vi "Write Source Waveform Task Data Property.vi"(8 "error in (no error)":errorcluster, 10 "Source Waveform Data":T2, 11 "Result Section ref":T1=18446744073709551615 format="%.0x") -> (0 "error out":errorcluster, 3 "Result Section ref out":T1=18446744073709551615 format="%.0x")   [LabVIEW 2015, in "Waveform-Processing-Custom-Device System Explorer.lvlib"]
uses:
  Waveform-Processing-Custom-Device System Explorer.lvlib
  <vilib>/NI Veristand/Custom Device API/Custom Device Item Ref.ctl
  Shared/Constants.vi
  <vilib>/NI Veristand/Custom Device API/Set Item Property (Double).vi
  <vilib>/NI Veristand/Custom Device API/Set Item Property (Boolean).vi
  <vilib>/NI Veristand/Custom Device API/Set Item Property (U32).vi
  <vilib>/NI VeriStand/Custom Device API/Custom Device API.lvlib
  Shared/Waveform-Processing-Custom-Device Shared.lvlib
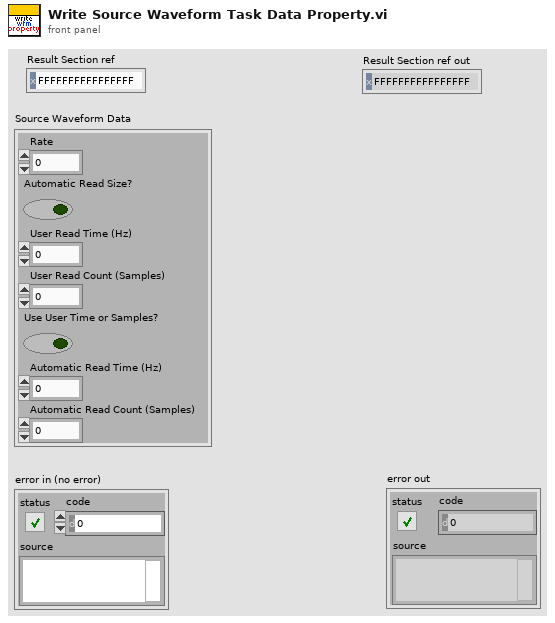
[diagram p1: front panel]
types:
  T1 = typedef "Custom Device API.lvlib/Custom Device Item Ref.ctl" = u64
  T2 = cluster{"Rate":dbl, "Automatic Read Size?":bool, "User Read Time (Hz) ":dbl, "User Read Count (Samples) ":u32, "Use User Time or Samples?":bool, "Automatic Read Time (Hz)":dbl, "Automatic Read Count (Samples)":u32}
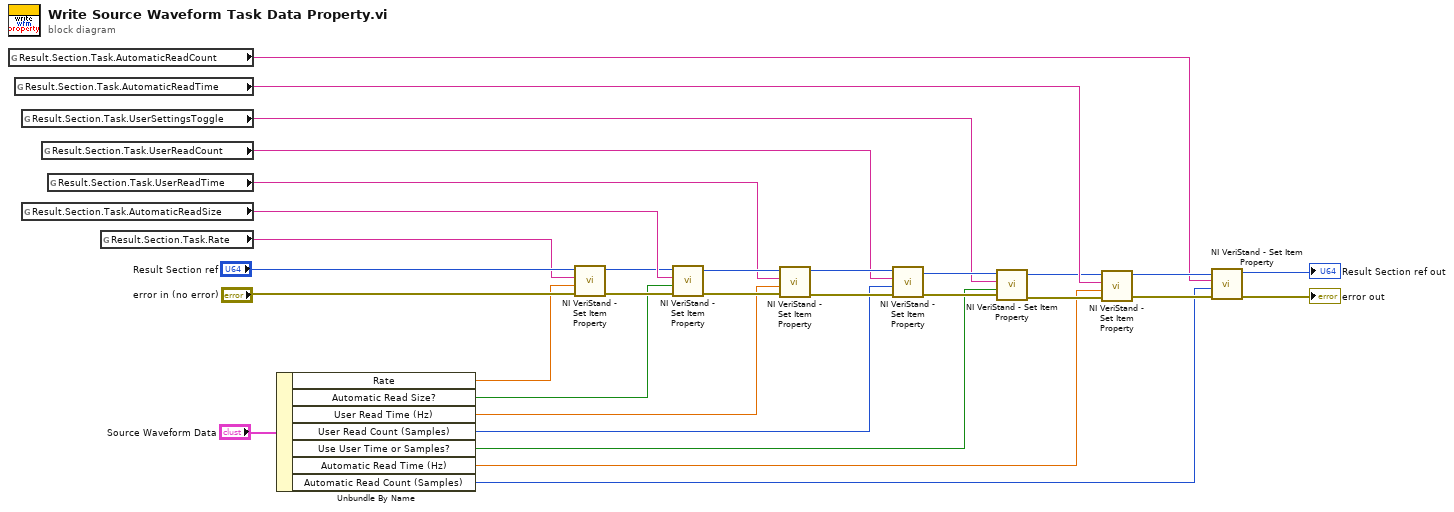
[diagram p0: block diagram]
diagram:
  n1 = global read "Constants.vi" "Result.Section.Task.AutomaticReadCount"() -> (w4:string)
  n2 = global read "Constants.vi" "Result.Section.Task.AutomaticReadTime"() -> (w10:string)
  n3 = global read "Constants.vi" "Result.Section.Task.UserSettingsToggle"() -> (w13:string)
  n4 = global read "Constants.vi" "Result.Section.Task.AutomaticReadSize"() -> (w26:string)
  n5 = global read "Constants.vi" "Result.Section.Task.UserReadCount"() -> (w16:string)
  n6 = global read "Constants.vi" "Result.Section.Task.UserReadTime"() -> (w20:string)
  n7 = global read "Constants.vi" "Result.Section.Task.Rate"() -> (w28:string)
  n8 = Unbundle By Name("Source Waveform Data") -> ("Rate"=w27:dbl, "Automatic Read Size?"=w23:bool, "User Read Time (Hz)"=w19:dbl, "User Read Count (Samples)"=w12:u32, "Use User Time or Samples?"=w11:bool, "Automatic Read Time (Hz)"=w7:dbl, "Automatic Read Count (Samples)"=w3:u32)
  n9 = call-poly <vilib>:"NI VeriStand - Set Item Property.vi"("error in (no error)"="error in (no error)", "Value"=w27, "Property Name"=w28, "Item Ref in"="Result Section ref") -> ("error out"=w25:errorcluster, "Item Ref out"=w24:T1)  [unwired: 5 in, 1 out]
  n10 = call-poly <vilib>:"NI VeriStand - Set Item Property.vi"("error in (no error)"=w25, "Value"=w23, "Property Name"=w26, "Item Ref in"=w24) -> ("error out"=w22:errorcluster, "Item Ref out"=w21:T1)  [unwired: 5 in, 1 out]
  n11 = call-poly <vilib>:"NI VeriStand - Set Item Property.vi"("error in (no error)"=w22, "Value"=w19, "Property Name"=w20, "Item Ref in"=w21) -> ("error out"=w18:errorcluster, "Item Ref out"=w17:T1)  [unwired: 5 in, 1 out]
  n12 = call-poly <vilib>:"NI VeriStand - Set Item Property.vi"("error in (no error)"=w18, "Value"=w12, "Property Name"=w16, "Item Ref in"=w17) -> ("error out"=w15:errorcluster, "Item Ref out"=w14:T1)  [unwired: 5 in, 1 out]
  n13 = call-poly <vilib>:"NI VeriStand - Set Item Property.vi"("error in (no error)"=w15, "Value"=w11, "Property Name"=w13, "Item Ref in"=w14) -> ("error out"=w8:errorcluster, "Item Ref out"=w9:T1)  [unwired: 5 in, 1 out]
  n14 = call-poly <vilib>:"NI VeriStand - Set Item Property.vi"("error in (no error)"=w8, "Value"=w7, "Property Name"=w10, "Item Ref in"=w9) -> ("error out"=w5:errorcluster, "Item Ref out"=w6:T1)  [unwired: 5 in, 1 out]
  n15 = call-poly <vilib>:"NI VeriStand - Set Item Property.vi"("error in (no error)"=w5, "Value"=w3, "Property Name"=w4, "Item Ref in"=w6) -> ("error out"=→"error out":errorcluster, "Item Ref out"=→"Result Section ref out":T1)  [unwired: 5 in, 1 out]
